vi "getDiagnosticResults.vi"(0 "connection ID":refnum<k5>, 1 "axis":i32, 5 "error":errorcluster) -> (14 "connection ID out":refnum<k5>, 15 "axis_out":i32, 16 "capacity":i32, 17 "resistance":i32, 19 "error out":errorcluster)   [LabVIEW 2016, in "amc_api.lvlib"]
doc: "Returns the results of the last diagnostic run and an error, if there was no run, it is currently running or the run failed"
uses:
  amc_api.lvlib
panel:
  out "jsonRespIn":string
  out "JSON-response":string="{\"jsonrpc\":\"2.0\",\"method\":\"\",\"params\":[5,1.245,true,\"name\"],\"id\":\"1\"}"
  out "JSON request":string
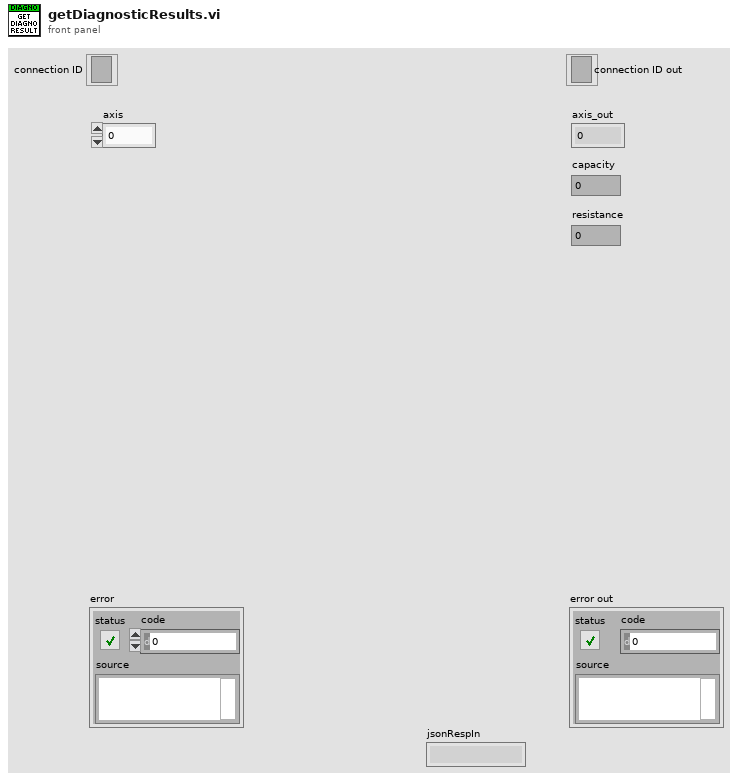
[diagram p1: front panel]
types:
  T1 = cluster{"jsonrpc":string, "method":string, "params":string[], "id":string, "api":i32, "pid":string}
  T2 = enum16{"Standard", "Buffered", "CRLF", "Immediate"}
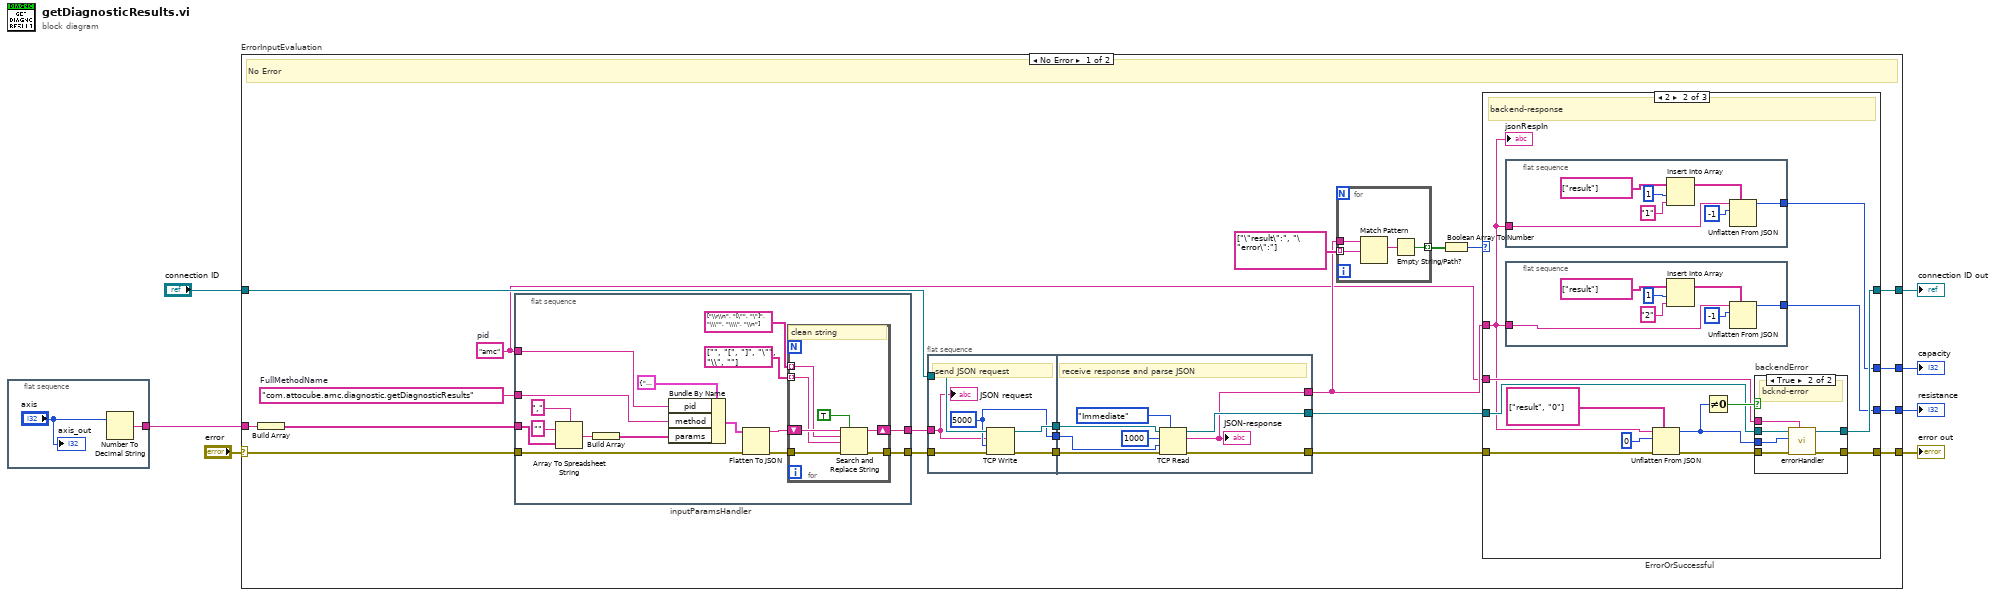
[diagram p0: block diagram]
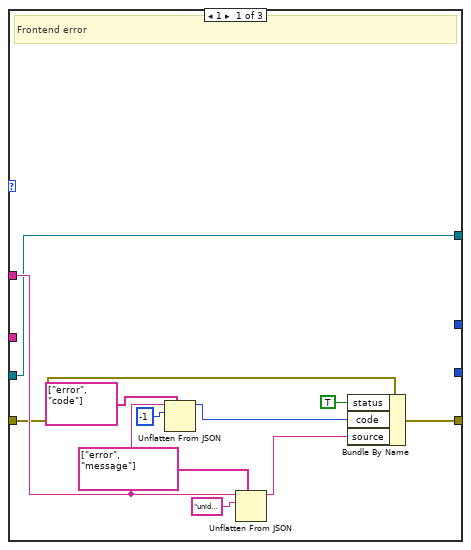
[diagram p2: hidden frame]
diagram:
  n1 = flat-sequence "in_axis" {
    tunnel: [w9] -> w3
    frame #0 {
      n2 = Number To Decimal String(number="axis") -> (decimal integer string=w9:string)  [unwired: 1 in]
      "axis_out" <- "axis"
    }
  }
  n3 = case "ErrorInputEvaluation" shown="No Error" "error" {
    selector: "error" -> [w23 w120]
    tunnel: "connection ID" -> [w27 w121]
    tunnel: [w14 w120] -> w6
    tunnel: [w15 w121] -> w5
    tunnel: w3 -> [w12 _]
    tunnel: [w11 _] -> w2
    tunnel: [w10 _] -> w1
    frame No Error {
      w13 = "amc"  # pid
      w24 = "com.attocube.amc.diagnostic.getDiagnosticResults"  # FullMethodName
      # "No Error"
      n4 = Build Array ("ParametersArrayString")(w12) -> (w22:string[])
      n5 = flat-sequence "inputParamsHandler" {
        tunnel: [w84] -> w21
        tunnel: w22 -> [w90]
        tunnel: w23 -> [w89]
        tunnel: [w86] -> w20
        tunnel: w24 -> [w80]
        tunnel: w13 -> [w79]
        frame #0 {
          n6 = Array To Spreadsheet String(delimiter (Tab)=",", array=w90, 3:"" ("format string")) -> (spreadsheet string=w92:string)
          n7 = Build Array "Build Array"(w92) -> (w81:string[])
          n8 = Bundle By Name(cluster=T1 {"jsonrpc"="2.0", "method"="com.attocube.amc.res.setRESReadOutFreq", "params"=[], "id"="1", "api"=2, "pid"=""} ("Cluster"), "pid"=w79, "method"=w80, "params"=w81) -> (w91:T1)
          n9 = Flatten To JSON(anything=w91, error in (no error)=w89) -> (JSON string=w85:string, 11:w87:errorcluster)  [unwired: 1 in]
          n10 = for {
            tunnel: string[] ["\\r\\n", "[\"", "\"]", "\\\"", "\\\\", "\\n"] ("search string") -> [w98] mode=indexing
            tunnel: string[] ["", "[", "]", "\"", "\\", ""] ("replace string (\"\")") -> [w97] mode=indexing
            shift-right: [w100] -> w84
            shift-left: w85 -> [w99]
            tunnel: w87 -> [w96]
            tunnel: [w95] -> w86
            # "clean string"
            n11 = Search and Replace String(replace all?=TRUE ("replace all? (F)"), input string=w99, search string=w98, replace string=w97, error in=w96) -> (result string=w100:string, error out=w95:errorcluster)  [unwired: 3 in, 2 out]
          }
        }
      }
      n12 = flat-sequence {
        tunnel: w27 -> [w111]
        tunnel: [w109] -> w30
        tunnel: [w110] -> w29
        tunnel: w20 -> [w106]
        tunnel: [w108] -> w28
        tunnel: w21 -> [w107]
        tunnel: [w115] -> w19
        tunnel: w30 -> [w117]
        tunnel: w29 -> [w116]
        tunnel: [w113] -> w18
        tunnel: w28 -> [w114]
        tunnel: [w112] -> w17
        frame #0 {
          w108 = 5000 ("timeout ms (25000)")
          # "send JSON request"
          n13 = TCP Write(connection ID=w111, data in=w107, error in (no error)=w106, 9:w108) -> (connection ID out=w109:refnum<k5>, error out=w110:errorcluster)  [unwired: 1 out]
          "JSON request" <- w107
        }
        frame #1 {
          # "receive response and parse JSON"
          n14 = TCP Read(connection ID=w117, bytes to read=1000, error in (no error)=w116, 7:T2."Immediate" ("mode (standard)"), 9:w114) -> (connection ID out=w115:refnum<k5>, data out=w112:string, error out=w113:errorcluster)
          "JSON-response" <- w112
        }
      }
      n15 = for {
        tunnel: string[] ["\"result\":", "\"error\":"] ("path") -> [w104] mode=indexing
        tunnel: [w102] -> w25 mode=indexing
        tunnel: w17 -> [w105]
        n16 = Match Pattern(string=w105, regular expression=w104) -> (match substring=w103:string)  [unwired: 1 in, 3 out]
        n17 = Empty String/Path?(string/path=w103) -> (empty?=w102:bool)
      }
      n18 = Boolean Array To Number(Boolean array=w25) -> (number=w16:u32)
      n19 = case "ErrorOrSuccessful" shown="2" w16 {
        tunnel: w17 -> [w33 w46 _]
        tunnel: w19 -> [w31 w48 w78]
        tunnel: [w31 w47 w78] -> w15
        tunnel: [w34 w44 w77] -> w14
        tunnel: w18 -> [w32 w45 w77]
        tunnel: w13 -> [_ w49 _]
        tunnel: [_ w43 _] -> w11
        tunnel: [_ w42 _] -> w10
        frame 1 {
          # "Frontend error"
          n20 = Unflatten From JSON(path=string[] ["error", "code"], JSON string=w33, type and defaults=-1) -> (value=w40:i32)  [unwired: 4 in, 1 out]
          n21 = Unflatten From JSON(path=string[] ["error", "message"], JSON string=w33, type and defaults="unidentified error") -> (value=w41:string)  [unwired: 4 in, 1 out]
          n22 = Bundle By Name(cluster=w32, "status"=TRUE, "code"=w40, "source"=w41) -> (w34:errorcluster)
        }
        frame 2 {
          # "backend-response"
          n23 = flat-sequence "out_integer" {
            tunnel: w46 -> [w64]
            tunnel: [w62] -> w43
            frame #0 {
              n24 = Insert Into Array(array=string[] ["result"] ("path"), index=1, new element="1" ("idx")) -> (w66:string[])
              n25 = Unflatten From JSON(path=w66, JSON string=w64, type and defaults=-1 ("index")) -> (value=w62:i32)  [unwired: 4 in, 1 out]
            }
          }
          n26 = flat-sequence "out_integer" {
            tunnel: w46 -> [w57]
            tunnel: [w55] -> w42
            frame #0 {
              n27 = Insert Into Array(array=string[] ["result"] ("path"), index=1, new element="2" ("idx")) -> (w59:string[])
              n28 = Unflatten From JSON(path=w59, JSON string=w57, type and defaults=-1 ("index")) -> (value=w55:i32)  [unwired: 4 in, 1 out]
            }
          }
          n29 = Unflatten From JSON(path=string[] ["result", "0"], JSON string=w46, type and defaults=0, error in (no error)=w45) -> (value=w50:i32, error out=w52:errorcluster)  [unwired: 3 in]
          n30 = Not Equal To 0?(x=w50) -> (x != 0?=w51:bool)
          n31 = case "backendError" shown="True" w51 {
            tunnel: w50 -> [_ w76]
            tunnel: w52 -> [w70 w75]
            tunnel: [w69 w74] -> w47
            tunnel: [w70 w73] -> w44
            tunnel: w48 -> [w69 w72]
            tunnel: w49 -> [_ w71]
            frame False {
              # "successful"
            }
            frame True {
              # "bcknd-error"
              n32 = call "errorHandler.vi"("pid"=w71, "error in"=w75, "errNbr"=w76, "connection ID"=w72) -> ("error out 2"=w73:errorcluster, "connection ID out"=w74:refnum<k5>)  [unwired: 6 in]
            }
          }
          "jsonRespIn" <- w46
        }
        frame Default {
          # "NoResponse"
        }
      }
    }
    frame Error {
      # "Error"
    }
  }
  "error out" <- w6
  "connection ID out" <- w5
  "capacity" <- w2
  "resistance" <- w1
